vi "Process Write Request.vi"(8 "error in (no error)":errorcluster, 10 "Write Request":refnum<class "WriteRequest.lvclass">, 11 "ConnectionManager in":refnum<class "ConnectionManager.lvclass">) -> (0 "error out":errorcluster, 3 "ConnectionManager out":refnum<class "ConnectionManager.lvclass">)   [LabVIEW 2019, in "ConnectionManager.lvlib" / "ConnectionManager.lvclass"]
uses:
  <vilib>/gpm_packages/@cs/Network-interface/Source/ConnectionManager/ConnectionManager/ConnectionManager.lvclass
  C:/Program Files/National Instruments/LabVIEW 2019/vi.lib/gpm_packages/@cs/Network-interface/Source/Logged Actor/LoggedActor.lvclass
  <vilib>/gpm_packages/@cs/Network-interface/Source/MessagingInterfaces/WriteRequest/WriteRequest.lvclass
  <vilib>/gpm_packages/@cs/Network-interface/Source/ConnectionManager/ConnectionManager/ConnectionManager.lvclass/ConnectionManager.ctl
  <vilib>/gpm_packages/@cs/event-logger/Source/Composed Log/Types/Log Level.ctl
  <vilib>/gpm_packages/@cs/Network-interface/Source/Logged Actor/LoggedActor.lvclass/LoggedActor.ctl
  <vilib>/gpm_packages/@cs/event-logger/Source/Composed Log/LoggerReference/LoggerReference.lvclass/LoggerReference.ctl
  <vilib>/gpm_packages/@cs/event-logger/Source/Composed Log/LoggerReference/Log Event.vi
  <vilib>/gpm_packages/@cs/event-logger/Source/Composed Log/LoggerReference/Log.vi
  <vilib>/gpm_packages/@cs/event-logger/Source/Composed Log/LoggerReference/Get Valid Event Time.vi
  <vilib>/gpm_packages/@cs/event-logger/Source/Composed Log/LoggerReference/Remove Stale Logs.vi
  <vilib>/gpm_packages/@cs/Network-interface/Source/Logged Actor/LoggedActor.lvclass
  <vilib>/gpm_packages/@cs/event-logger/Source/Composed Log/Composed Log.lvlib
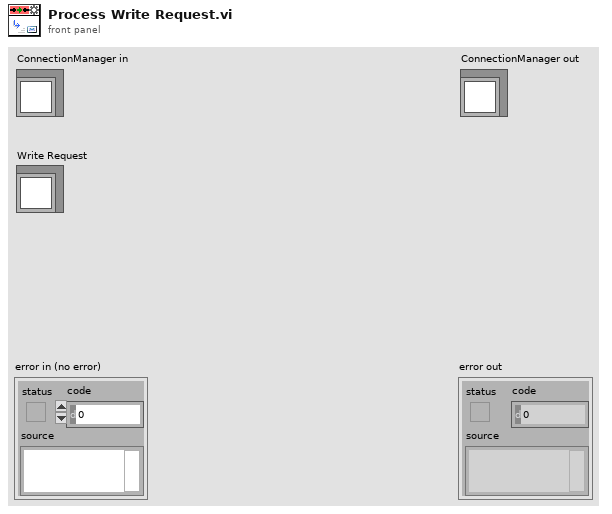
[diagram p1: front panel]
types:
  T1 = typedef "Composed Log.lvlib/Log Level.ctl" = enum16{"Debug", "Info", "Warning", "Error", "Critical"}
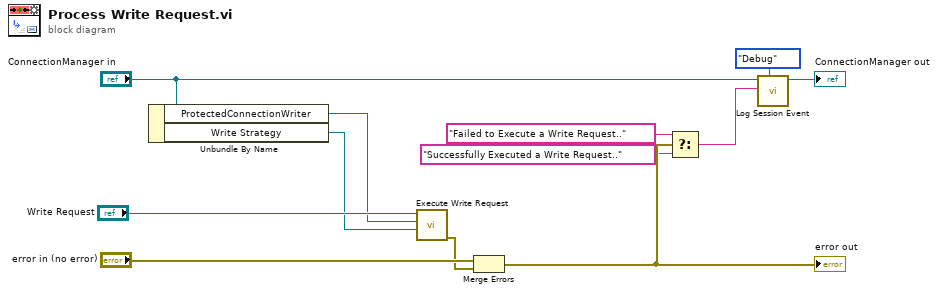
[diagram p0: block diagram]
diagram:
  n1 = Unbundle By Name("ConnectionManager in") -> ("ProtectedConnectionWriter"=w11:refnum<class "ProtectedConnectionWriter.lvclass">, "Write Strategy"=w10:refnum<class "IWriteStrategy.lvclass">)
  n2 = call-dynamic "Execute Write Request.vi"("IWritePolicy in"=w10, "Connection Writer"=w11, "WriteRequest in"="Write Request") -> ("error out"=w8:errorcluster)  [unwired: 8 in]
  n3 = Merge Errors("error in (no error)", w8) -> (w4:errorcluster)
  "error out" <- w4
  n4 = Select(t="Failed to Execute a Write Request..", s=w4, f="Successfully Executed a Write Request..") -> (s? t:f=w2:string)
  n5 = call <vilib>:"Log Session Event.vi"("Event Level"=Log_Level."Debug", "Event Data"=w2, "SessionActor in"="ConnectionManager in") -> ("SessionActor out"=→"ConnectionManager out":refnum<class "ConnectionManager.lvclass">)  [unwired: 7 in, 1 out]
